vi "Shock_Capture_Rev.B.vi"() -> ()   [LabVIEW 2017]
uses:
  <vilib>/express/express analysis/Spectral/Block/exnSpectralBlock spectral measurements PSD poly.vi
  <vilib>/express/express analysis/Spectral/Block/exnSpectralBlock spectral measurements PSD DDT.vi
  <vilib>/express/express analysis/Spectral/XNode/ExpressSpectralMeasurementsBlockNode.xnode
panel:
  out "Data Recording":bool
  out "DAQ Error":string=" INSTRUCTIONS:\r\rNormal Use:  When using subVIs that incorporate the error in/error out (or error I/O) structure, place this handler where you want to inform the user of an error, typically at the end of the I/O data path, as the last action of the program.  If the error in error? is ERROR, the handler creates a message describing the error and its source.  If the type of dialog = 1 (default), the message is displayed to the user, who can only acknowedge it.  If the type = 2, the user can acknowledge the message or abort execution; aborting a program with active I/O is not recommended.  If the type = 0, no message is displayed; this is used to process the error programmatically, and the error out cluster elements are wired to individual terminals for that reason.  \r\rOther Use:\n\r\nlocal testing.  To test the error code of a subVI or function that does not have the error I/O structure, you can wire its error code and a source string to the local error code and error source inputs.  If error in error? indicates no error and error code is not equal to 0, the local code and source are substituted for the error in values, and error? is set TRUE (ERROR)."
  out "PSD Error":string=" INSTRUCTIONS:\r\rNormal Use:  When using subVIs that incorporate the error in/error out (or error I/O) structure, place this handler where you want to inform the user of an error, typically at the end of the I/O data path, as the last action of the program.  If the error in error? is ERROR, the handler creates a message describing the error and its source.  If the type of dialog = 1 (default), the message is displayed to the user, who can only acknowedge it.  If the type = 2, the user can acknowledge the message or abort execution; aborting a program with active I/O is not recommended.  If the type = 0, no message is displayed; this is used to process the error programmatically, and the error out cluster elements are wired to individual terminals for that reason.  \r\rOther Use:\n\r\nlocal testing.  To test the error code of a subVI or function that does not have the error I/O structure, you can wire its error code and a source string to the local error code and error source inputs.  If error in error? indicates no error and error code is not equal to 0, the local code and source are substituted for the error in values, and error? is set TRUE (ERROR)."
  out "Minimum 2":dbl
  out "Maximum 2":dbl
  out "RMS 2":dbl
  out "Minimum":dbl
  out "Maximum":dbl
  out "RMS":dbl
  out "Waveform Graph":dynamicdata(graph)
  in  "Stop":bool
  out "Time History":dynamicdata(graph)
  # "Shock Data Capture VI"
  # "Accelerometer 1"
  # "Accelerometer 2"
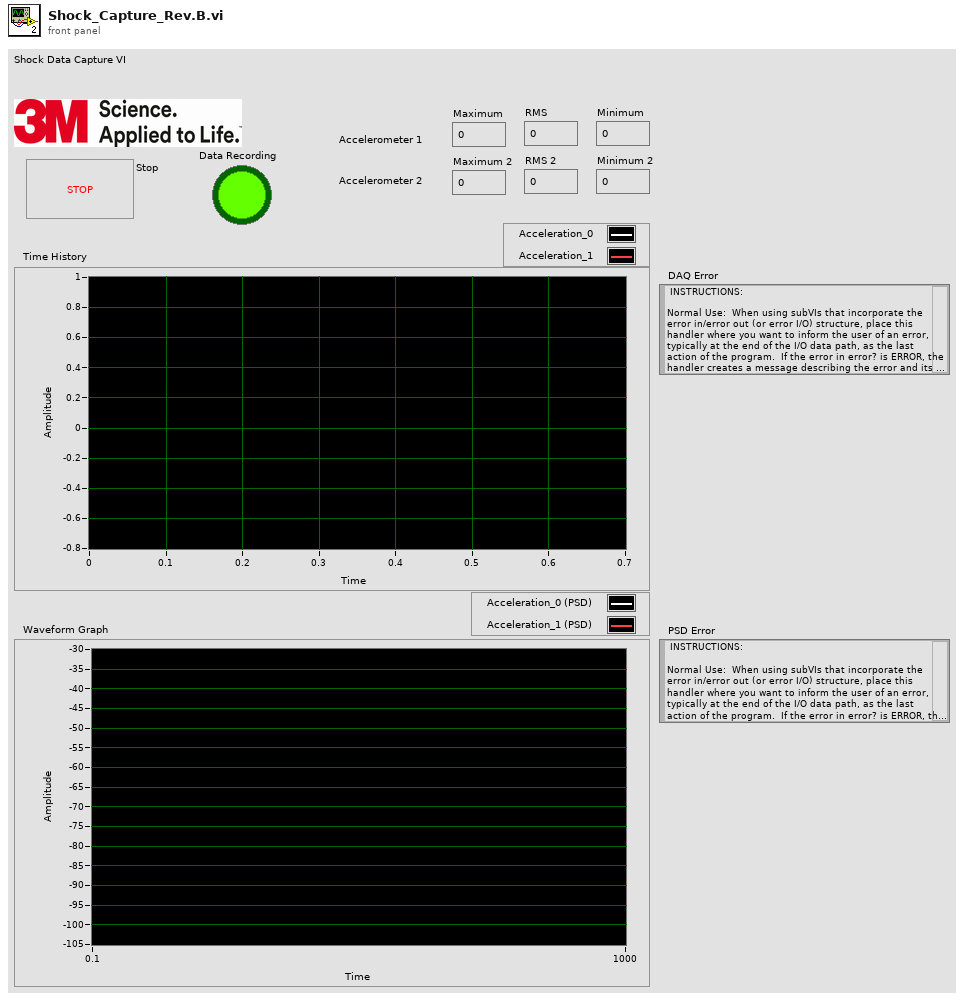
[diagram p1: front panel]
types:
  T1 = cluster{"averaging mode":u16, "weighting mode":u16, "number of averages":u32}
  T2 = cluster{"dB On (F)":bool, "unwrap phase (F)":bool, "convert to degree (F)":bool}
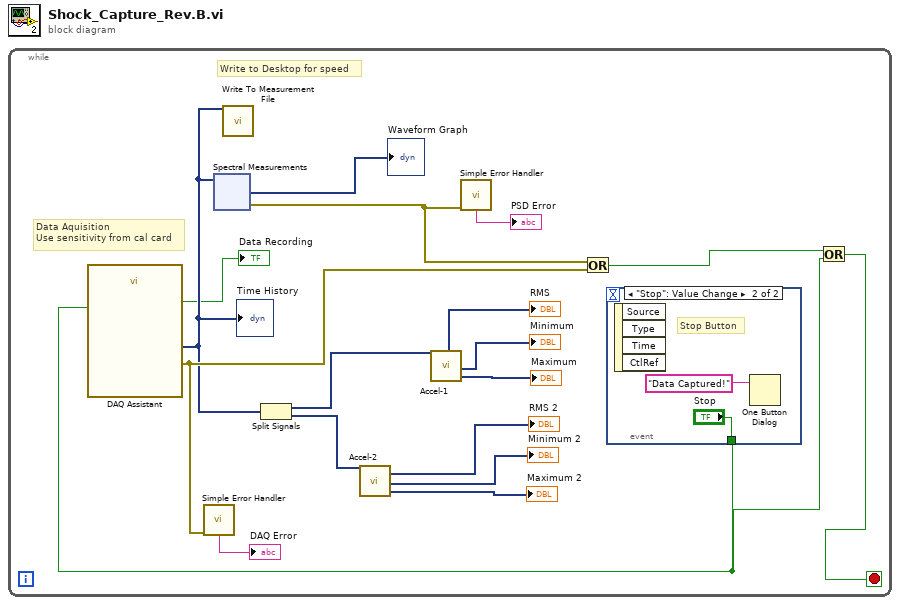
[diagram p0: block diagram]
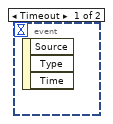
[diagram p2: hidden frame]
diagram:
  n1 = while {
    stop <- w3 stop-if-true
    # "Write to Desktop for speed"
    # "Data Aquisition\nUse sensitivity from cal card"
    n2 = event shown="[1] \"Stop\": Value Change" {
      selector: _ -> [_ _]
      dyn-events: _ -> [_ _]
      timeout: _ -> [_ _]
      tunnel: [_ "Stop"] -> w1
      event Timeout {
        n3 = event-data() -> ()  [unwired: 1 in, 3 out]
      }
      event "Stop": Value Change {
        # "Stop Button"
        n4 = event-data() -> ()  [unwired: 1 in, 4 out]
        n5 = One Button Dialog(message="Data Captured!") -> ()  [unwired: 1 in, 1 out]
      }
    }
    n6 = call "DAQ Assistant"("stop (F)"=w1) -> ("data"=w6:dynamicdata, "stopped"=→"Data Recording":bool, "error out"=w14:errorcluster)  [unwired: 15 in, 1 out]
    "Time History" <- w6
    n7 = call <vilib>:"Simple Error Handler.vi"("error in (no error)"=w14) -> ("message"=→"DAQ Error":string)  [unwired: 4 in, 4 out]
    n8 = xnode "Spectral Measurements"("Signals"=w6) -> ("PSD"=→"Waveform Graph":dynamicdata, "error out"=w5:errorcluster)  [unwired: 1 in]
    n9 = call "Write To Measurement File"("Signals"=w6) -> ()  [unwired: 16 in, 3 out]
    n10 = Split Signals(w6) -> (w7:dynamicdata, w13:dynamicdata)  [unwired: 2 in]
    n11 = call "Accel-2"("Signals"=w13) -> ("RMS"=→"RMS 2":dynamicdata, "Minimum"=→"Minimum 2":dynamicdata, "Maximum"=→"Maximum 2":dynamicdata)  [unwired: 22 in, 2 out]
    n12 = call "Accel-1"("Signals"=w7) -> ("RMS"=→"RMS":dynamicdata, "Minimum"=→"Minimum":dynamicdata, "Maximum"=→"Maximum":dynamicdata)  [unwired: 22 in, 2 out]
    n13 = call <vilib>:"Simple Error Handler.vi"("error in (no error)"=w5) -> ("message"=→"PSD Error":string)  [unwired: 4 in, 4 out]
    n14 = Or(x=w5, y=w14) -> (x .or. y?=w12:bool)
    n15 = Or(x=w12, y=w1) -> (x .or. y?=w3:bool)
  }
